vi "Example Callback - TiltState Callback.vi"(4 "TiltState":refnum<user-event>, 5 "Event Data":cluster{"sender":refnum<k24>, "state":u8}, 6 "Control Ref":refnum<k24>, 7 "Event Common Data":T1) -> ()   [LabVIEW 2013]
uses:
  C:/tf/play/labview/Tinkerforge.dll
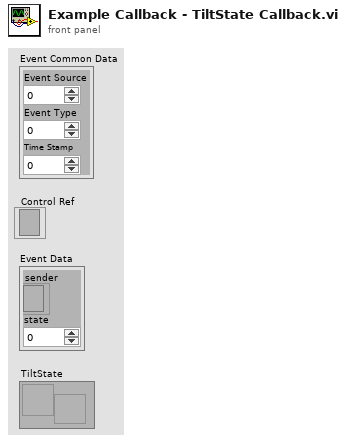
[diagram p1: front panel]
types:
  T1 = cluster{"Event Source":i32, "Event Type":u32, "Time Stamp":u32}
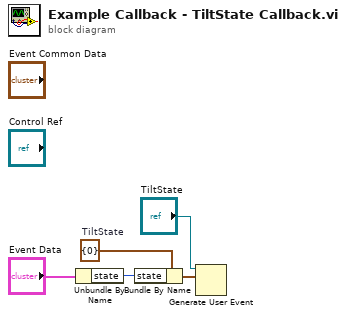
[diagram p0: block diagram]
diagram:
  w3 = cluster{"state":u8} {"state"=0}  # TiltState
  n1 = Unbundle By Name("Event Data") -> ("state"=w4:u8)
  n2 = Bundle By Name(cluster=w3, "state"=w4) -> (w2:cluster{"state":u8})
  n3 = Generate User Event(user event="TiltState", event data cluster=w2) -> ()  [unwired: 2 in, 2 out]
